vi "Escape Non Displayable Characters.vi"(11 "Raw String":string) -> (3 "Escaped String":string)   [LabVIEW 2020, in "Reports.lvlib" / "XML Report.lvclass"]
uses:
  XML Report.lvclass
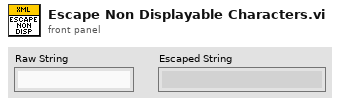
[diagram p1: front panel]
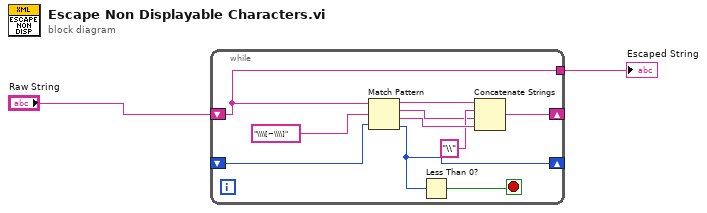
[diagram p0: block diagram]
diagram:
  n1 = while {
    shift-right: [w3] -> _
    shift-left: "Raw String" -> [w4]
    shift-right: [w7] -> _
    shift-left: _ -> [w6]
    tunnel: [w4] -> w1
    stop <- w5 stop-if-true
    n2 = Match Pattern(string=w4, regular expression="\\\\[~\\\\]", offset (0)=w6) -> (before substring=w12:string, match substring=w8:string, after substring=w11:string, offset past match=w7:i32)
    n3 = Less Than 0?(x=w7) -> (x < 0?=w5:bool)
    n4 = Concatenate Strings(w12, "\\" ("replace string (\"\")"), w8, w11) -> (w3:string)
  }
  "Escaped String" <- w1
